vi "Generate Rake Maps.vi"(8 "error in (no error)":errorcluster, 10 "Auto Release Amount of Lines in Rake (Enabled)":bool, 11 "Amount of Lines in Rake":refnum<class "1D Array s32.lvclass">) -> (0 "error out":errorcluster, 1 "Rake Keys":refnum<class "2D Array u32.lvclass">, 2 "In Bounds Mask":refnum<class "2D Array binary.lvclass">, 3 "Line Indexes":refnum<class "2D Array f32.lvclass">, 5 "Line Divisions":refnum<class "1D Array f32.lvclass">)   [LabVIEW 2020, in "G2CPU Line Profile.lvlib"]
uses:
  G2CPU Line Profile.lvlib
  <vilib>/Natan Biesmans/G2CPU GPU and CPU HPC Toolkit/G2CPU Libraries/Arrays/1DArray/s32/1D Array s32.lvclass
  C:/Program Files/National Instruments/LabVIEW 2025/vi.lib/Natan Biesmans/G2CPU GPU and CPU HPC Toolkit/G2CPU Libraries/Arrays/Array/Array Prototype.lvclass
  <vilib>/Natan Biesmans/G2CPU GPU and CPU HPC Toolkit/G2CPU Libraries/Arrays/2DArray/u32/2D Array u32.lvclass
  <vilib>/Natan Biesmans/G2CPU GPU and CPU HPC Toolkit/G2CPU Libraries/Arrays/2DArray/binary/2D Array binary.lvclass
  <vilib>/Natan Biesmans/G2CPU GPU and CPU HPC Toolkit/G2CPU Libraries/Arrays/2DArray/f32/2D Array f32.lvclass
  <vilib>/Natan Biesmans/G2CPU GPU and CPU HPC Toolkit/G2CPU Libraries/Arrays/1DArray/f32/1D Array f32.lvclass
  <vilib>/Natan Biesmans/G2CPU GPU and CPU HPC Toolkit/G2CPU Libraries/Arrays/Array/Array Prototype.lvclass/Array Prototype.ctl
  5d478299-bdbd-4f87-896c-a179d6b9d395.vi
  2d17aa69-f9fe-4b17-9b2f-b7e58b045a88.vi
  f403d4df-35fe-4b95-8300-4ee0e84e63b8.vi
  8f89d022-d2c4-4576-bb01-3eb29fe3eb3d.vi
  a0e39a42-1683-4516-87fc-062200535f8c.vi
  fbbde881-12b3-465d-aca1-0d9fc1832a11.vi
  a3b473a8-4a02-4593-89ec-f7a88b3d702a.vi
  a921baa9-a1c1-42d1-a6fe-f604268927c7.vi
  <vilib>/Natan Biesmans/G2CPU GPU and CPU HPC Toolkit/G2CPU Libraries/Arrays/Array/G2CPU Get Array Pointer.vi
  5d478299-bdbd-4f87-896c-a179d6b9d395.vi/72eb0651-ae32-4ba2-a447-070823507cb2.vi
  2d17aa69-f9fe-4b17-9b2f-b7e58b045a88.vi/e7247370-a01f-465a-ac0e-4dfefcb1bb87.vi
  2d17aa69-f9fe-4b17-9b2f-b7e58b045a88.vi/345e91f0-9a5e-4de4-af9c-133346717e4a.vi
  f403d4df-35fe-4b95-8300-4ee0e84e63b8.vi/ab6cfe59-c8ad-4da3-839b-8d02ec9e015f.vi
  8f89d022-d2c4-4576-bb01-3eb29fe3eb3d.vi/ab6cfe59-c8ad-4da3-839b-8d02ec9e015f.vi
  a0e39a42-1683-4516-87fc-062200535f8c.vi/cfed8f62-9c64-4dab-912e-5e7c21cb720b.vi
  fbbde881-12b3-465d-aca1-0d9fc1832a11.vi/5793b77b-c002-4ebf-9075-685617c95341.vi
  fbbde881-12b3-465d-aca1-0d9fc1832a11.vi/2ed3ef86-c00d-4d71-b84c-20267a6dfcf9.vi
  a3b473a8-4a02-4593-89ec-f7a88b3d702a.vi/2cbae9c5-d993-4013-91e6-67de96abb5a0.vi
  a3b473a8-4a02-4593-89ec-f7a88b3d702a.vi/df7b902d-6356-419a-b5d5-2ac54df1e506.vi
  a921baa9-a1c1-42d1-a6fe-f604268927c7.vi/1bf6e03b-eb75-45f6-9764-49dc38a3a024.vi
  a921baa9-a1c1-42d1-a6fe-f604268927c7.vi/2da4419f-02df-47a7-be00-1b7e0871fa33.vi
  f403d4df-35fe-4b95-8300-4ee0e84e63b8.vi/ab6cfe59-c8ad-4da3-839b-8d02ec9e015f.vi/313ec8c5-c203-475c-9de0-0583f6fb8b4d.vi
  8f89d022-d2c4-4576-bb01-3eb29fe3eb3d.vi/ab6cfe59-c8ad-4da3-839b-8d02ec9e015f.vi/313ec8c5-c203-475c-9de0-0583f6fb8b4d.vi
  a0e39a42-1683-4516-87fc-062200535f8c.vi/cfed8f62-9c64-4dab-912e-5e7c21cb720b.vi/77c7badc-ed81-4514-99c1-20d37f4e5ecc.vi
  a0e39a42-1683-4516-87fc-062200535f8c.vi/cfed8f62-9c64-4dab-912e-5e7c21cb720b.vi/eb76fa01-6782-47b4-b34f-9eb474c9cc78.vi
  <vilib>/Natan Biesmans/G2CPU GPU and CPU HPC Toolkit/ArrayFire Driver/VIs/Run as Multi Device.vi
  fbbde881-12b3-465d-aca1-0d9fc1832a11.vi/5793b77b-c002-4ebf-9075-685617c95341.vi/3e802c67-fb96-46a3-ae13-4994a8508b4f.vi
  fbbde881-12b3-465d-aca1-0d9fc1832a11.vi/5793b77b-c002-4ebf-9075-685617c95341.vi/5a50fc67-79e7-4972-80c2-92243cd53dd4.vi
  fbbde881-12b3-465d-aca1-0d9fc1832a11.vi/2ed3ef86-c00d-4d71-b84c-20267a6dfcf9.vi/730f6c57-5c0b-4ee9-b61e-75067b25222b.vi
  fbbde881-12b3-465d-aca1-0d9fc1832a11.vi/2ed3ef86-c00d-4d71-b84c-20267a6dfcf9.vi/096b8799-7810-404e-baca-ba9279cec4bd.vi
  fbbde881-12b3-465d-aca1-0d9fc1832a11.vi/2ed3ef86-c00d-4d71-b84c-20267a6dfcf9.vi/0f1a5a47-bcc5-4796-ac31-8dfcfbc0d7d1.vi
  fbbde881-12b3-465d-aca1-0d9fc1832a11.vi/2ed3ef86-c00d-4d71-b84c-20267a6dfcf9.vi/89f12e17-3330-4b72-ad8f-8dd636660732.vi
  a3b473a8-4a02-4593-89ec-f7a88b3d702a.vi/df7b902d-6356-419a-b5d5-2ac54df1e506.vi/edd31282-7992-4bba-af75-482693dee5e1.vi
  a921baa9-a1c1-42d1-a6fe-f604268927c7.vi/1bf6e03b-eb75-45f6-9764-49dc38a3a024.vi/3e802c67-fb96-46a3-ae13-4994a8508b4f.vi
  a921baa9-a1c1-42d1-a6fe-f604268927c7.vi/1bf6e03b-eb75-45f6-9764-49dc38a3a024.vi/5a50fc67-79e7-4972-80c2-92243cd53dd4.vi
  a921baa9-a1c1-42d1-a6fe-f604268927c7.vi/1bf6e03b-eb75-45f6-9764-49dc38a3a024.vi/4b7910ad-0c4a-46e4-b1b3-c9721aeaa91e.vi
  a921baa9-a1c1-42d1-a6fe-f604268927c7.vi/2da4419f-02df-47a7-be00-1b7e0871fa33.vi/730f6c57-5c0b-4ee9-b61e-75067b25222b.vi
  a921baa9-a1c1-42d1-a6fe-f604268927c7.vi/2da4419f-02df-47a7-be00-1b7e0871fa33.vi/096b8799-7810-404e-baca-ba9279cec4bd.vi
  a921baa9-a1c1-42d1-a6fe-f604268927c7.vi/2da4419f-02df-47a7-be00-1b7e0871fa33.vi/0f1a5a47-bcc5-4796-ac31-8dfcfbc0d7d1.vi
  a921baa9-a1c1-42d1-a6fe-f604268927c7.vi/2da4419f-02df-47a7-be00-1b7e0871fa33.vi/89f12e17-3330-4b72-ad8f-8dd636660732.vi
  a921baa9-a1c1-42d1-a6fe-f604268927c7.vi/1bf6e03b-eb75-45f6-9764-49dc38a3a024.vi/5a50fc67-79e7-4972-80c2-92243cd53dd4.vi/1b7cf390-2ae0-48f3-9bce-03c57eed6ee8.vi
  <vilib>/Natan Biesmans/G2CPU GPU and CPU HPC Toolkit/ArrayFire Driver/VIs/max all.vi
  <vilib>/Natan Biesmans/G2CPU GPU and CPU HPC Toolkit/G2CPU Libraries/Arrays/Array/G2CPU Release Array.vi
  <vilib>/Natan Biesmans/G2CPU GPU and CPU HPC Toolkit/ArrayFire Driver/VIs/cast.vi
  <vilib>/Natan Biesmans/G2CPU GPU and CPU HPC Toolkit/G2CPU Libraries/Arrays/Array/G2CPU Set Array Pointer.vi
  <vilib>/Natan Biesmans/G2CPU GPU and CPU HPC Toolkit/ArrayFire Driver/VIs/range.vi
  <vilib>/Natan Biesmans/G2CPU GPU and CPU HPC Toolkit/ArrayFire Driver/VIs/iszero.vi
  <vilib>/Natan Biesmans/G2CPU GPU and CPU HPC Toolkit/ArrayFire Driver/VIs/sub.vi
  <vilib>/Natan Biesmans/G2CPU GPU and CPU HPC Toolkit/ArrayFire Driver/VIs/release array.vi
  <vilib>/Natan Biesmans/G2CPU GPU and CPU HPC Toolkit/ArrayFire Driver/subvi/Error Converter (ErrCode or Status).vi
  <vilib>/Natan Biesmans/G2CPU GPU and CPU HPC Toolkit/ArrayFire Driver/VIs/add.vi
  <vilib>/Natan Biesmans/G2CPU GPU and CPU HPC Toolkit/G2CPU Libraries/Arrays/SubVI/is 2D.vi
  <vilib>/Natan Biesmans/G2CPU GPU and CPU HPC Toolkit/ArrayFire Driver/VIs/lt.vi
  <vilib>/Natan Biesmans/G2CPU GPU and CPU HPC Toolkit/G2CPU Libraries/Arrays/SubVI/is 1D.vi
  <vilib>/Natan Biesmans/G2CPU GPU and CPU HPC Toolkit/G2CPU Libraries/Arrays/Array/Array Prototype.lvclass
  <vilib>/Natan Biesmans/G2CPU GPU and CPU HPC Toolkit/G2CPU Libraries/Arrays/1DArray/1D Array Prototype.lvclass
  <vilib>/Natan Biesmans/G2CPU GPU and CPU HPC Toolkit/G2CPU Libraries/Arrays/2DArray/2D Array Prototype.lvclass
  <vilib>/Natan Biesmans/G2CPU GPU and CPU HPC Toolkit/G2CPU Libraries/Arrays/DataTypes/f32/f32.lvclass
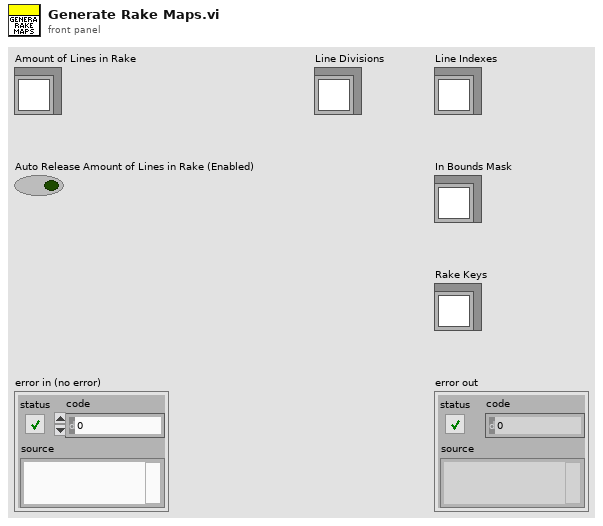
[diagram p1: front panel]
types:
  T1 = typedef "AF.lvlib/Dim4.ctl" = cluster{"Dim 0":u64, "Dim 1":u64, "Dim 2":u64, "Dim 3":u64}
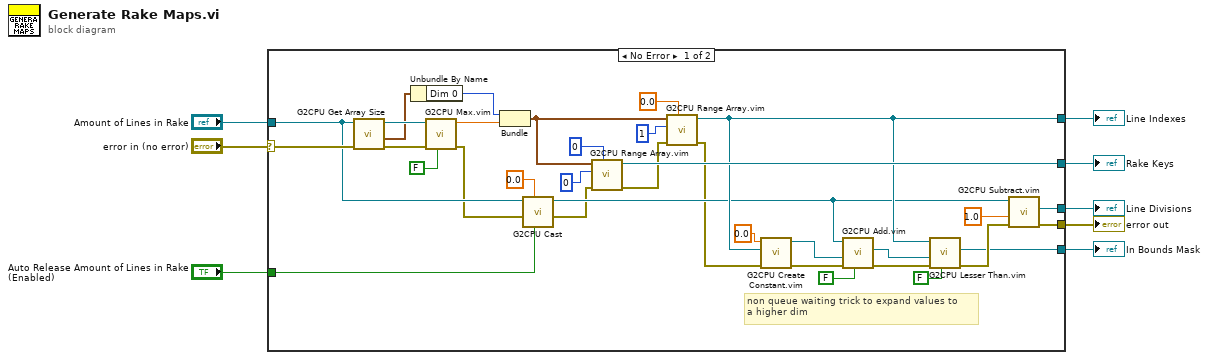
[diagram p0: block diagram]
diagram:
  n1 = case shown="No Error" "error in (no error)" {
    selector: "error in (no error)" -> [w40 w43]
    tunnel: [w42 w43] -> w8
    tunnel: "Amount of Lines in Rake" -> [w39 _]
    tunnel: [w37 _] -> w4
    tunnel: [w36 _] -> w3
    tunnel: [w34 _] -> w2
    tunnel: [w33 _] -> w1
    tunnel: "Auto Release Amount of Lines in Rake (Enabled)" -> [w41 _]
    frame No Error {
      # "non queue waiting trick to expand values to\na higher dim"
      n2 = call <vilib>:"G2CPU Get Array Size.vi"("error in (no error)"=w40, "Array in"=w39) -> ("error out"=w18:errorcluster, "Array Size"=w17:T1, "Array out"=w19:refnum<class "1D Array s32.lvclass">)  [unwired: 6 in, 1 out]
      n3 = Unbundle By Name(w17) -> ("Dim 0"=w29:u64)
      n4 = call "G2CPU Max.vim"("Auto Release (Enabled)"=FALSE, "error in (no error)"=w18, "Array First"=w19) -> ("error out"=w25:errorcluster, "real out"=w28:dbl)  [unwired: 6 in, 1 out]
      n5 = Bundle("Dim 0"=w29, "real out"=w28) -> (w22:cluster{"Dim 0":u64, "real out":dbl})  [unwired: 1 in]
      n6 = call "G2CPU Cast"("Auto Release Low (Enabled)"=w41, "Datatype Prototype"=sgl 0.0 ("single precision float"), "error in (no error)"=w25, "Array In"=w39) -> ("error out"=w21:errorcluster, "Array Out"=w32:refnum<class "1D Array f32.lvclass">)  [unwired: 6 in]
      n7 = call "G2CPU Range Array.vim"("Datatype"=u32 0, "Error in"=w21, "Sequential Dimension"=0, "Size"=w22) -> ("error out"=w20:errorcluster, "Array out"=w37:refnum<class "2D Array u32.lvclass">)  [unwired: 6 in]
      n8 = call "G2CPU Range Array.vim"("Datatype"=sgl 0.0, "Error in"=w20, "Sequential Dimension"=1, "Size"=w22) -> ("error out"=w15:errorcluster, "Array out"=w34:refnum<class "2D Array f32.lvclass">)  [unwired: 6 in]
      n9 = call "G2CPU Create Constant.vim"("error in (no error)"=w15, "Size"=w34, "val"=sgl 0.0) -> ("error out"=w14:errorcluster, "object out"=w12:refnum<class "2D Array f32.lvclass">)  [unwired: 7 in]
      n10 = call "G2CPU Add.vim"("Auto Release lhs (Enabled)"=FALSE, "error in (no error)"=w14, "Array rhs"=w12, "Array lhs"=w32) -> ("error out"=w13:errorcluster, "Array Result"=w11:refnum<class "2D Array f32.lvclass">)  [unwired: 6 in]
      n11 = call "G2CPU Lesser Than.vim"("Auto Release lhs (Enabled)"=FALSE, "error in (no error)"=w13, "Array rhs"=w11, "Array lhs"=w34) -> ("error out"=w38:errorcluster, "Array Result"=w36:refnum<class "2D Array binary.lvclass">)  [unwired: 6 in]
      n12 = call "G2CPU Subtract.vim"("error in (no error)"=w38, "Array rhs"=sgl 1.0 ("Datatype"), "Array lhs"=w32) -> ("error out"=w42:errorcluster, "Array Result"=w33:refnum<class "1D Array f32.lvclass">)  [unwired: 7 in]
    }
    frame Error {
    }
  }
  "error out" <- w8
  "Rake Keys" <- w4
  "In Bounds Mask" <- w3
  "Line Indexes" <- w2
  "Line Divisions" <- w1
